vi "perform asynchronous fault handling.vi"(0 "module in":T5, 1 "worker pool reference":T1, 2 "error classification":T4, 3 "iteration":u64, 5 "module ref in":refnum<data-value>, 7 "code":i32, 9 "fault handling in":T6, 11 "run flags in":u8, 12 "engine error in":errorcluster, 13 "engine reference":i32, 14 "cfg ref":refnum<data-value>) -> (4 "module out":T5, 6 "go to safe state":bool, 8 "code out":i32, 10 "engine error out":errorcluster, 15 "run flags out":u8)   [LabVIEW 2013, in "main engine.lvlib"]
uses:
  main engine.lvlib
  fault handling spec.ctl
  Configuration/Error Actions.ctl
  <vilib>/NI/Tag Bus Module Framework/runtime/TBM module execution interface.lvclass
  async executor/asynchronous executor reference.ctl
  async executor/message to executor.ctl
  Runtime/async command notification.ctl
  <vilib>/NI/Tag Bus/table/data table.ctl
  Runtime/async error info.ctl
  <vilib>/NI/Tag Bus Module Framework/runtime/error classification.ctl
  <vilib>/NI/Tag Bus Module Framework/module configuration/TBM module configuration.lvclass
  worker library/worker comms.ctl
  worker library/worker commands.ctl
  worker library/request fifos.ctl
  worker library/recovery request.ctl
  worker library/rt fault.ctl
  worker library/response fifos.ctl
  worker library/recovery response.ctl
  <vilib>/NI/Module Execution Interface/Engine Runtime/Fault.ctl
  worker library/worker pool.lvlib
  Configuration/Standard Engine Configuration.lvclass
  <vilib>/NI/Tag Bus/table/data table.lvlib
  async executor/async executor.lvlib
  <vilib>/NI/Module Execution Interface/Engine Runtime/Engine Runtime Interface.lvclass
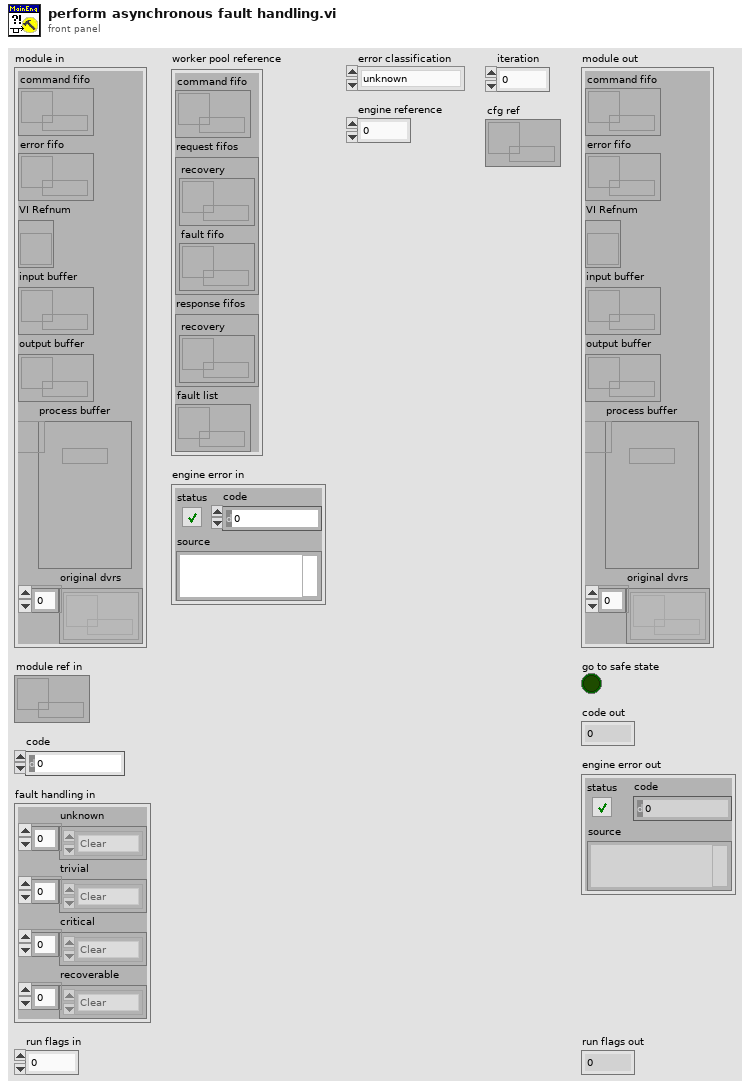
[diagram p1: front panel]
types:
  T1 = typedef "worker pool.lvlib/worker comms.ctl" = cluster{"command fifo":refnum<k33>, "request fifos":T2, "response fifos":T3, "fault list":refnum<data-value>}
  T2 = typedef "worker pool.lvlib/request fifos.ctl" = cluster{"recovery":refnum<k33>, "fault fifo":refnum<k33>}
  T3 = typedef "worker pool.lvlib/response fifos.ctl" = cluster{"recovery":refnum<k33>}
  T4 = typedef "TBM module execution interface.lvclass/error classification.ctl" = enum16{"unknown", "none", "trivial", "recoverable", "critical"}
  T5 = typedef "async executor.lvlib/asynchronous executor reference.ctl" = cluster{"command fifo":refnum<k33>, "error fifo":refnum<k33>, "VI Refnum":refnum<vi>, "input buffer":refnum<k33>, "output buffer":refnum<k33>, "process buffer":refnum<k33>, "original dvrs":refnum<data-value>[]}
  T6 = typedef "main engine.lvlib/fault handling spec.ctl" = cluster{"unknown":T7[], "trivial":T7[], "critical":T7[], "recoverable":T7[]}
  T7 = typedef "Standard Engine Configuration.lvclass/Error Actions.ctl" = enum16{"Clear", "Notify", "Stop Component", "Stop Engine", "Safe State", "Attempt Recovery"}
  T8 = typedef "worker pool.lvlib/rt fault.ctl" = cluster{"code":i32, "classification":T4, "iteration":u64, "cfg ref":refnum<data-value>}
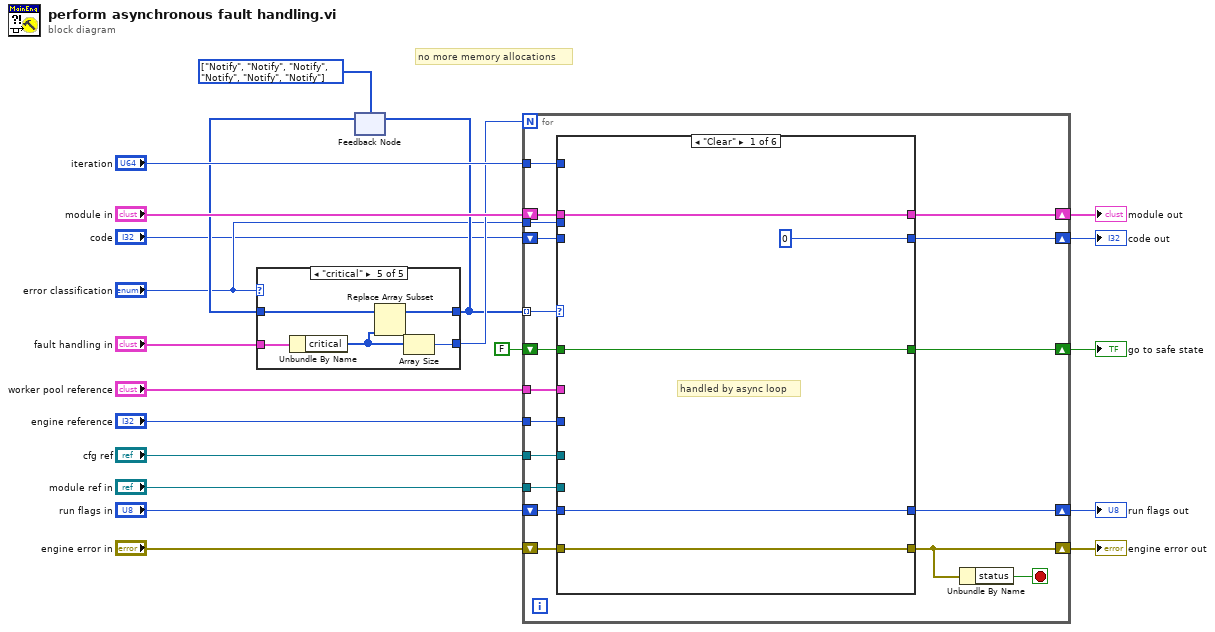
[diagram p0: block diagram]
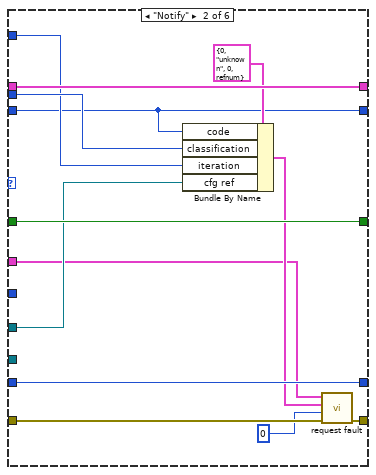
[diagram p2: hidden frame]
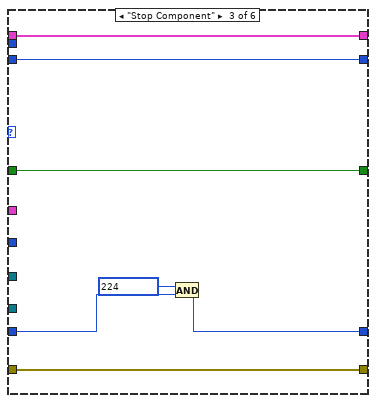
[diagram p3: hidden frame]
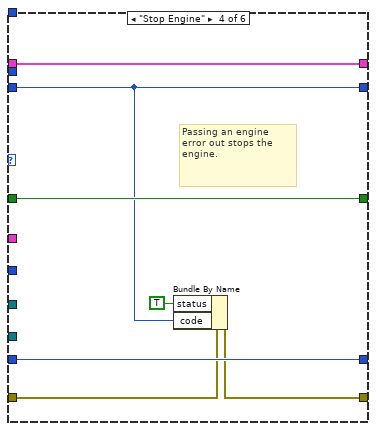
[diagram p4: hidden frame]
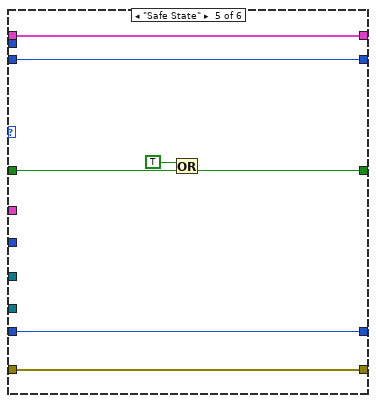
[diagram p5: hidden frame]
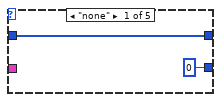
[diagram p7: hidden frame]
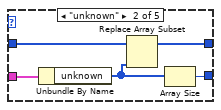
[diagram p8: hidden frame]
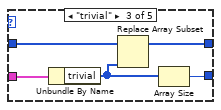
[diagram p9: hidden frame]
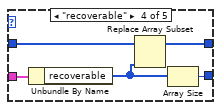
[diagram p10: hidden frame]
diagram:
  w5 = T7[] [enum."Notify", enum."Notify", enum."Notify", enum."Notify", enum."Notify", enum."Notify"] items=["Clear", "Notify", "Stop Component", "Stop Engine", "Safe State", "Attempt Recovery"] ("critical")
  # "no more memory allocations"
  n1 = feedback #1(w5) -> (w6:T7[])
  n2 = case shown="\"critical\"" "error classification" {
    tunnel: "fault handling in" -> [_ w28 w33 w38 w43]
    tunnel: [w22 w25 w30 w35 w40] -> w7
    tunnel: [0 w27 w32 w37 w42] -> w8
    tunnel: w6 -> [w22 w26 w31 w36 w41]
    frame "none" {
    }
    frame "unknown" {
      n3 = Unbundle By Name(w28) -> ("unknown"=w24:T7[])
      n4 = Replace Array Subset(array=w26, new element=w24) -> (w25:T7[])  [unwired: 1 in]
      n5 = Array Size(array=w24) -> (size(s)=w27:i32)
    }
    frame "trivial" {
      n6 = Unbundle By Name(w33) -> ("trivial"=w29:T7[])
      n7 = Replace Array Subset(array=w31, new element=w29) -> (w30:T7[])  [unwired: 1 in]
      n8 = Array Size(array=w29) -> (size(s)=w32:i32)
    }
    frame "recoverable" {
      n9 = Unbundle By Name(w38) -> ("recoverable"=w34:T7[])
      n10 = Replace Array Subset(array=w36, new element=w34) -> (w35:T7[])  [unwired: 1 in]
      n11 = Array Size(array=w34) -> (size(s)=w37:i32)
    }
    frame "critical" {
      n12 = Unbundle By Name(w43) -> ("critical"=w39:T7[])
      n13 = Replace Array Subset(array=w41, new element=w39) -> (w40:T7[])  [unwired: 1 in]
      n14 = Array Size(array=w39) -> (size(s)=w42:i32)
    }
  }
  n15 = feedback-in #1(w7) -> ()
  n16 = for {
    N: w8 -> [_]
    shift-right: [w54] -> w16
    shift-left: "run flags in" -> [w55]
    shift-right: [w57] -> w2
    shift-left: "code" -> [w58]
    shift-right: [w60] -> w17
    shift-left: "module in" -> [w59]
    tunnel: "worker pool reference" -> [w51]
    tunnel: w7 -> [w61] mode=indexing
    shift-right: [w52] -> w14
    shift-left: "engine error in" -> [w53]
    tunnel: "error classification" -> [w50]
    tunnel: "iteration" -> [w49]
    shift-right: [w48] -> w11
    shift-left: FALSE -> [w47]
    tunnel: "cfg ref" -> [w46]
    tunnel: "module ref in" -> [w56]
    tunnel: "engine reference" -> [w45]
    stop <- w44 stop-if-true
    n17 = case shown="\"Clear\"" w61 {
      tunnel: [w63 w79 w86 w93 w100 w101] -> w60
      tunnel: w59 -> [w63 w79 w86 w93 w100 w101]
      tunnel: w58 -> [_ w72 w85 w87 w99 w105]
      tunnel: [0 ("code") w72 w85 w87 w99 w105] -> w57
      tunnel: w56 -> [_ _ _ _ _ _]
      tunnel: w55 -> [w66 w78 w84 w92 w98 w103]
      tunnel: [w66 w78 w81 w92 w98 w103] -> w54
      tunnel: w53 -> [w65 w70 w83 w89 w97 w102]
      tunnel: [w65 w71 w83 w90 w97 w102] -> w52
      tunnel: w51 -> [_ w68 _ _ _ _]
      tunnel: w50 -> [_ w76 _ _ _ _]
      tunnel: w49 -> [_ w75 _ _ _ _]
      tunnel: [w64 w74 w82 w91 w95 w104] -> w48
      tunnel: w47 -> [w64 w74 w82 w91 w96 w104]
      tunnel: w46 -> [_ w73 _ _ _ _]
      tunnel: w45 -> [_ _ _ _ _ _]
      frame "Clear" {
        # "handled by async loop"
      }
      frame "Notify" {
        n18 = Bundle By Name(cluster=T8 {"code"=0, "classification"=enum."unknown", "iteration"=0, "cfg ref"=refnum} ("element"), "code"=w72, "classification"=w76, "iteration"=w75, "cfg ref"=w73) -> (w69:T8)
        n19 = call "request fault.vi"("error in"=w70, "timeout in ms (0)"=0, "rt fault"=w69, "worker comms in"=w68) -> ("error out"=w71:errorcluster)  [unwired: 7 in]
      }
      frame "Stop Component" {
        n20 = And(x=u8 224, y=w84) -> (x .and. y?=w81:u8)
      }
      frame "Stop Engine" {
        # "Passing an engine error out stops the engine."
        n21 = Bundle By Name(cluster=w89, "status"=TRUE, "code"=w87) -> (w90:errorcluster)
      }
      frame "Safe State" {
        n22 = Or(x=TRUE, y=w96) -> (x .or. y?=w95:bool)
      }
      frame "Attempt Recovery" {
        # "handled by async"
      }
    }
    n23 = Unbundle By Name(w52) -> ("status"=w44:bool)
  }
  "module out" <- w17
  "run flags out" <- w16
  "engine error out" <- w14
  "go to safe state" <- w11
  "code out" <- w2
